vi "Agilent N6900 N7900 Series Output Volt Step Transient.vi"() -> ()   [LabVIEW 2021]
doc: "This example sets the power suppply to one voltage level for a certain amount of time, then steps to another voltage level for a certain amount of time, and then stops the output."
uses:
  <instrlib>/Agilent N6900 N7900 Series/Agilent N6900 N7900 Series.lvlib
panel:
  in  "Voltage Priority Current Upper Limit (2.50A)":dbl=2.5
  in  "Voltage Priority Current Lower Limit (-2.50A)":dbl=-2.5
  in  "Voltage Triggered Amplitude (0 V)":dbl
  in  "Voltage Immediate Amplitude (0 V)":dbl
  in  "Time After Step (10s)":dbl=10.0
  in  "Time Before Step (10s)":dbl=10.0
  in  "VISA resource name":refnum<visa-resource-name>
  # "(c) 2013-2018 National Instruments Corporation.  ALL RIGHTS RESERVED."
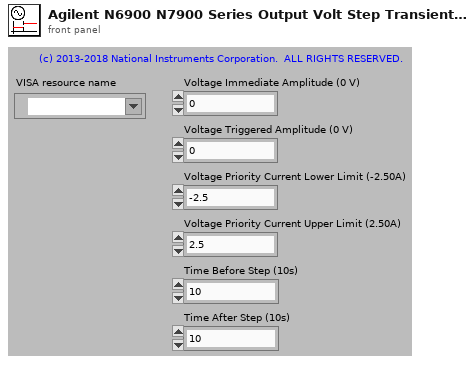
[diagram p1: front panel]
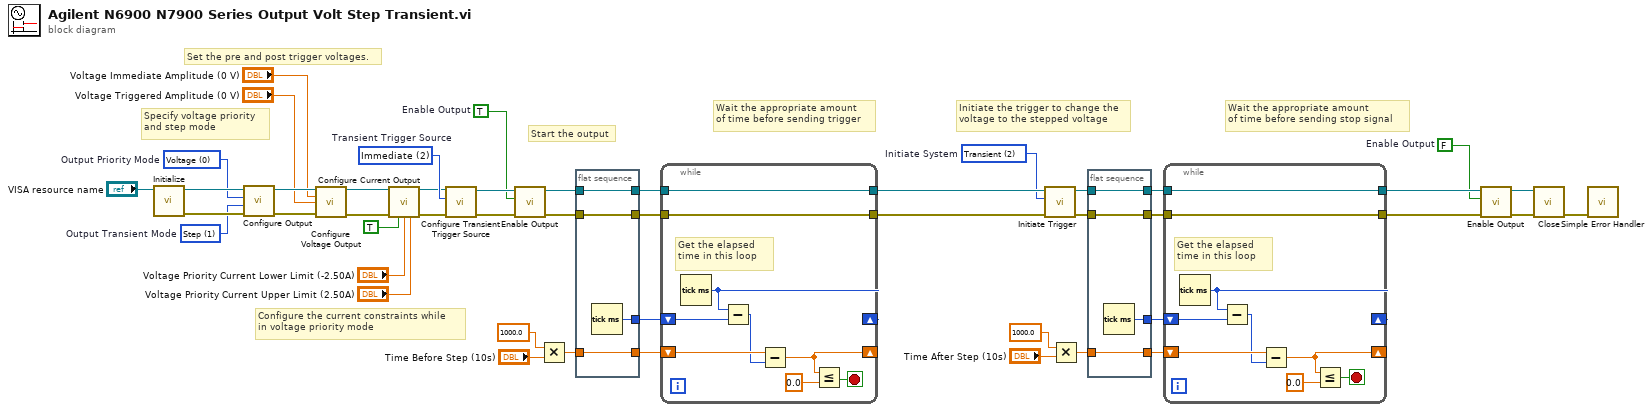
[diagram p0: block diagram]
diagram:
  w5 = FALSE  # Enable Output
  w10 = TRUE  # Enable Output
  w25 = u16 2 items=["Acquisition", "External Logging", "Transient"]  # Initiate System
  w41 = u16 2 items=["Bus", "External", "Immediate", "Pin 1", "Pin 2", "Pin 3", "Pin 4", "Pin 5", "Pin 6", "Pin 7"]  # Transient Trigger Source
  w28 = u16 0 items=["Voltage", "Current"]  # Output Priority Mode
  w29 = u16 1 items=["Fixed", "Step", "List", "Arbitrary"]  # Output Transient Mode
  # "Initiate the trigger to change the\nvoltage to the stepped voltage"
  # "Start the output"
  # "Specify voltage priority \nand step mode"
  # "Wait the appropriate amount\nof time before sending stop signal"
  # "Wait the appropriate amount\nof time before sending trigger"
  # "Configure the current constraints while\nin voltage priority mode"
  # "Set the pre and post trigger voltages."
  n1 = call <instrlib>:"Initialize.vi"("VISA resource name"="VISA resource name") -> ("error out"=w36:errorcluster, "VISA resource name out"=w37:refnum<visa-resource-name>)  [unwired: 9 in]
  n2 = call <instrlib>:"Configure Output.vi"("error in (no error)"=w36, "Output Transient Mode (0: Fixed)"=w29, "Output Priority Mode (0: Voltage)"=w28, "VISA resource name"=w37) -> ("error out"=w39:errorcluster, "VISA resource name out"=w38:refnum<visa-resource-name>)  [unwired: 6 in]
  n3 = call <instrlib>:"Configure Voltage Output.vi"("VISA resource name"=w38, "Voltage Immediate Amplitude (0 V)"="Voltage Immediate Amplitude (0 V)", "Voltage Triggered Amplitude (0 V)"="Voltage Triggered Amplitude (0 V)", "error in (no error)"=w39) -> ("VISA resource name out"=w12:refnum<visa-resource-name>, "error out"=w15:errorcluster)  [unwired: 10 in]
  n4 = call <instrlib>:"Configure Current Output.vi"("VISA resource name"=w12, "error in (no error)"=w15, "Enable Voltage Priority (False)"=TRUE ("Voltage Priority Enabled (False)"), "Voltage Priority Current Lower Limit (-2.50A)"="Voltage Priority Current Lower Limit (-2.50A)", "Voltage Priority Current Upper Limit (2.50A)"="Voltage Priority Current Upper Limit (2.50A)") -> ("VISA resource name out"=w13:refnum<visa-resource-name>, "error out"=w14:errorcluster)  [unwired: 9 in]
  n5 = call <instrlib>:"Configure Transient Trigger Source.vi"("error in (no error)"=w14, "Transient Trigger Source (0: Bus)"=w41, "VISA resource name"=w13) -> ("error out"=w34:errorcluster, "VISA resource name out"=w35:refnum<visa-resource-name>)  [unwired: 7 in]
  n6 = call <instrlib>:"Enable Output.vi"("error in (no error)"=w34, "Enable Output (F: Disable)"=w10, "VISA resource name"=w35) -> ("error out"=w31:errorcluster, "VISA resource name out"=w33:refnum<visa-resource-name>)  [unwired: 7 in]
  n7 = Multiply(x=1000.0, y="Time Before Step (10s)") -> (x*y=w42:dbl)
  n8 = flat-sequence {
    tunnel: [w51] -> w44
    tunnel: [w50] -> w43
    tunnel: w42 -> [w50]
    tunnel: w33 -> [w49]
    tunnel: [w49] -> w32
    tunnel: w31 -> [w48]
    tunnel: [w48] -> w30
    frame #0 {
      n9 = Tick Count (ms)() -> (millisecond timer value=w51:u32)
    }
  }
  n10 = while {
    shift-right: [w56] -> _
    shift-left: w43 -> [w58]
    shift-right: [w59] -> _
    shift-left: w44 -> [w60]
    tunnel: w32 -> [w52]
    tunnel: w30 -> [w53]
    tunnel: [w52] -> w27
    tunnel: [w53] -> w26
    stop <- w54 stop-if-true
    # "Get the elapsed time in this loop"
    n11 = Tick Count (ms)() -> (millisecond timer value=w59:u32)
    n12 = Subtract(x=w59, y=w60) -> (x-y=w57:u32)
    n13 = Subtract(x=w58, y=w57) -> (x-y=w56:dbl)
    n14 = Less Or Equal?(x=w56, y=0.0) -> (x <= y?=w54:bool)
  }
  n15 = call <instrlib>:"Initiate Trigger.vi"("error in (no error)"=w26, "Initiate System (0: Acquisition)"=w25, "VISA resource name"=w27) -> ("error out"=w20:errorcluster, "VISA resource name out"=w21:refnum<visa-resource-name>)  [unwired: 7 in]
  n16 = Multiply(x=1000.0, y="Time After Step (10s)") -> (x*y=w24:dbl)
  n17 = flat-sequence {
    tunnel: [w64] -> w22
    tunnel: [w63] -> w23
    tunnel: w24 -> [w63]
    tunnel: w21 -> [w62]
    tunnel: w20 -> [w61]
    tunnel: [w62] -> w19
    tunnel: [w61] -> w18
    frame #0 {
      n18 = Tick Count (ms)() -> (millisecond timer value=w64:u32)
    }
  }
  n19 = while {
    shift-right: [w69] -> _
    shift-left: w23 -> [w71]
    shift-right: [w72] -> _
    shift-left: w22 -> [w73]
    tunnel: w19 -> [w65]
    tunnel: w18 -> [w66]
    tunnel: [w66] -> w9
    tunnel: [w65] -> w8
    stop <- w67 stop-if-true
    # "Get the elapsed time in this loop"
    n20 = Tick Count (ms)() -> (millisecond timer value=w72:u32)
    n21 = Subtract(x=w72, y=w73) -> (x-y=w70:u32)
    n22 = Subtract(x=w71, y=w70) -> (x-y=w69:dbl)
    n23 = Less Or Equal?(x=w69, y=0.0) -> (x <= y?=w67:bool)
  }
  n24 = call <instrlib>:"Enable Output.vi"("error in (no error)"=w9, "Enable Output (F: Disable)"=w5, "VISA resource name"=w8) -> ("error out"=w7:errorcluster, "VISA resource name out"=w6:refnum<visa-resource-name>)  [unwired: 7 in]
  n25 = call <instrlib>:"Close.vi"("error in (no error)"=w7, "VISA resource name"=w6) -> ("error out"=w40:errorcluster)  [unwired: 9 in]
  n26 = call <vilib>:"Simple Error Handler.vi"("error in (no error)"=w40) -> ()  [unwired: 4 in, 5 out]
